vi "PPMS.getLHeLevel.vi"(8 "error in (no error)":errorcluster, 11 "instrument.PPMS":refnum<class "instrument.PPMS.lvclass">) -> (0 "error out":errorcluster, 2 "Helium Level (%)":dbl, 3 "instrument.PPMS out":refnum<class "instrument.PPMS.lvclass">)   [LabVIEW 2019, in "instrument.PPMS.lvclass"]
uses:
  instrument.PPMS.lvclass
  instrument.PPMS.lvclass/instrument.PPMS.ctl
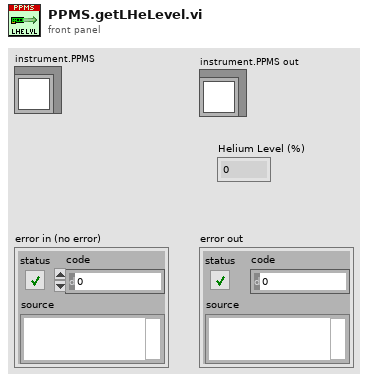
[diagram p1: front panel]
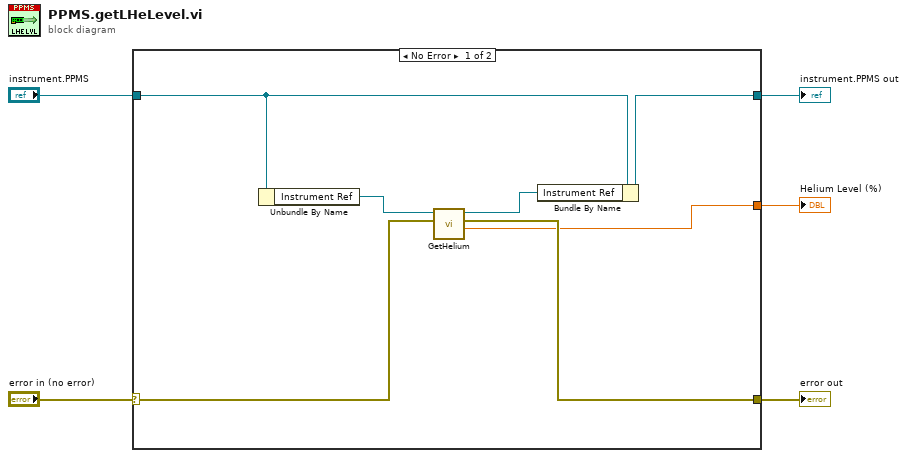
[diagram p0: block diagram]
diagram:
  n1 = case shown="No Error" "error in (no error)" {
    selector: "error in (no error)" -> [w11 w14]
    tunnel: [w10 w14] -> w5
    tunnel: "instrument.PPMS" -> [w6 w13]
    tunnel: [w7 w13] -> w2
    tunnel: [w9 _] -> w1
    frame No Error {
      n2 = Unbundle By Name(w6) -> ("Instrument Ref"=w12:refnum<k24>)
      n3 = call "GetHelium.vi"("error in (no error)"=w11, "Instrument Refnum in"=w12) -> ("Helium Level (%)"=w9:dbl, "error out"=w10:errorcluster, "Instrument Ref Out"=w8:refnum<k24>)  [unwired: 3 in]
      n4 = Bundle By Name(cluster=w6, "Instrument Ref"=w8) -> (w7:refnum<class "instrument.PPMS.lvclass">)
    }
    frame Error {
    }
  }
  "Helium Level (%)" <- w1
  "error out" <- w5
  "instrument.PPMS out" <- w2
